vi "Untitled 1.vi"   [LabVIEW 2018]
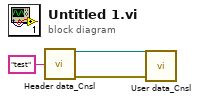
[diagram p0: block diagram]
diagram:
  n1 = call "Header data_Cnsl.vi"("file name"="test") -> ("refnum out"=w2:refnum<file>, "error out"=w1:errorcluster)  [unwired: 13 in]
  n2 = call "User data_Cnsl.vi"("Error In"=w1, "refnum in"=w2) -> ()  [unwired: 6 in, 2 out]
